vi "ClearCache.vi"(11 "inputs":string[](array[string])) -> (2 "output/failure":string, 3 "return code":i32)   [LabVIEW 2020]
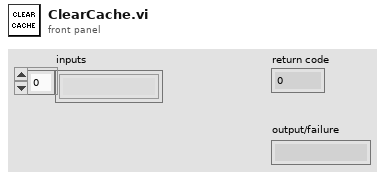
[diagram p1: front panel]
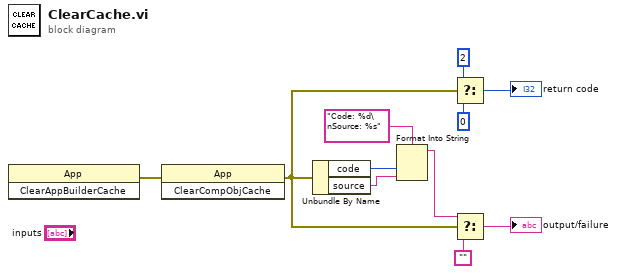
[diagram p0: block diagram]
diagram:
  n1 = invoke class="App" method="ClearAppBuilderCache"() -> (error out=w11:errorcluster)  [unwired: 3 in, 2 out]
  n2 = invoke class="App" method="ClearCompObjCache"(error in=w11) -> (error out=w7:errorcluster)  [unwired: 2 in, 2 out]
  n3 = Unbundle By Name(w7) -> ("code"=w6:i32, "source"=w5:string)
  n4 = Format Into String(format string="Code: %d\nSource: %s", w6, w5) -> (resulting string=w2:string)  [unwired: 2 in, 1 out]
  n5 = Select(t=2 ("return code"), s=w7, f=0 ("return code")) -> (s? t:f=→"return code":i32)
  n6 = Select(t=w2, s=w7, f="") -> (s? t:f=→"output/failure":string)
